vi "HistogramOfIntegers.vi"(0 "X":i32[](array[numeric]), 1 "intervals (unused)":i32=1) -> (2 "Histogram: h(x)":i32[](array[numeric]), 3 "X Values":i32[](array[numeric]), 4 "error":i32)   [LabVIEW 2011]
doc: "Finds the discrete histogram of the input sequence <B>X</B>."
panel:
  # "Histogram"
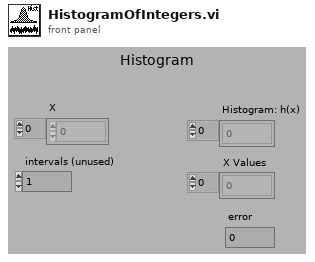
[diagram p1: front panel]
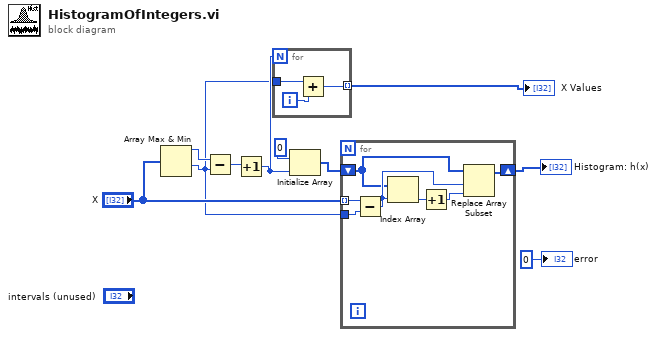
[diagram p0: block diagram]
diagram:
  n1 = Array Max & Min(array="X") -> (max value=w10:i32, min value=w3:i32)  [unwired: 2 out]
  n2 = Subtract(x=w10, y=w3) -> (x-y=w9:i32)
  n3 = Increment(x=w9) -> (x+1=w7:i32)
  n4 = for {
    N: w7 -> [_]
    tunnel: w3 -> [w12]
    tunnel: [w11] -> w6 mode=indexing
    i -> [w13]
    n5 = Add(x=w12, y=w13) -> (x+y=w11:i32)
  }
  "X Values" <- w6
  n6 = Initialize Array(0 ("element"), w7) -> (w4:i32[])
  n7 = for {
    tunnel: "X" -> [w20] mode=indexing
    shift-right: [w14] -> w2
    shift-left: w4 -> [w15]
    tunnel: w3 -> [w19]
    n8 = Subtract(x=w20, y=w19) -> (x-y=w16:i32)
    n9 = Index Array(array=w15, index=w16) -> (element=w17:i32)
    n10 = Increment(x=w17) -> (x+1=w18:i32)
    n11 = Replace Array Subset(array=w15, new element=w18, index=w16) -> (w14:i32[])
  }
  "Histogram: h(x)" <- w2
  "error" <- 0 ("error")
